vi "Read Static On.vi"(8 "error in (no error)":errorcluster, 11 "Meerstetter output in":refnum<class "Meerstetter output.lvclass">) -> (0 "error out":errorcluster, 2 "Static On":bool, 3 "Meerstetter output out":refnum<class "Meerstetter output.lvclass">)   [LabVIEW 2014, in "Meerstetter Lib.lvlib" / "Meerstetter output.lvclass"]
uses:
  Meerstetter output.lvclass
  Meerstetter output.lvclass/Meerstetter output.ctl
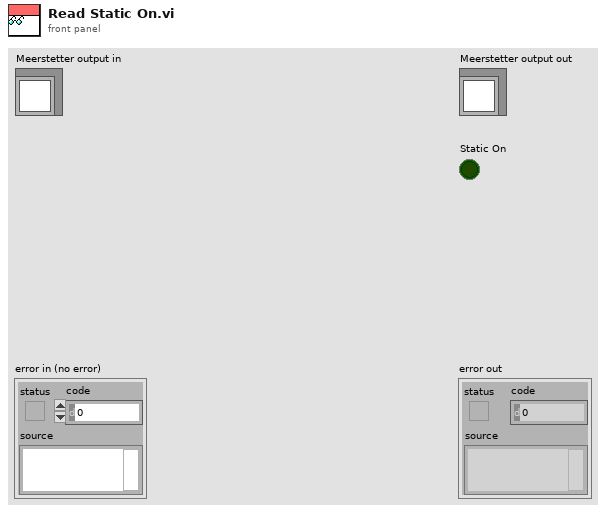
[diagram p1: front panel]
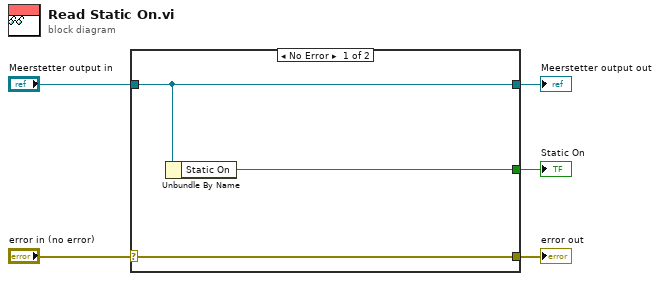
[diagram p0: block diagram]
diagram:
  n1 = case shown="No Error" "error in (no error)" {
    selector: "error in (no error)" -> [w8 w9]
    tunnel: [w8 w9] -> w4
    tunnel: [w7 w10] -> w2
    tunnel: "Meerstetter output in" -> [w7 w10]
    tunnel: [w6 _] -> w1
    frame No Error {
      n2 = Unbundle By Name(w7) -> ("Static On"=w6:bool)
    }
    frame Error {
    }
  }
  "error out" <- w4
  "Meerstetter output out" <- w2
  "Static On" <- w1
